vi "Stage Double Click.vi"(7 "Draw Area Size":T1, 8 "error in (no error)":errorcluster, 9 "Y (px)":i32, 10 "X (px)":i32, 11 "Application in":refnum<class "Application.lvclass">) -> (0 "error out":errorcluster, 3 "Application out":refnum<class "Application.lvclass">)   [LabVIEW 2023, in "Application.lvlib" / "Application.lvclass"]
uses:
  Application.lvclass
  Application.lvclass/Application.ctl
  Hardware/Stage Controller Messages/Move From Double Click Msg/Move From Double Click Msg.lvclass/Move From Double Click Msg.ctl
  <vilib>/ActorFramework/Message Enqueuer/Message Enqueuer.lvclass/Message Enqueuer.ctl
  <vilib>/ActorFramework/Message Enqueuer/Enqueue.vi
  Hardware/Stage Controller Messages/Move From Double Click Msg/Move From Double Click Msg.lvclass
  C:/Program Files/National Instruments/LabVIEW 2023/vi.lib/ActorFramework/Message/Message.lvclass
  <vilib>/ActorFramework/Message Priority Queue/Priority Enqueue.vi
  <vilib>/Utility/miscctls.llb/LVBoundsTypeDef.ctl
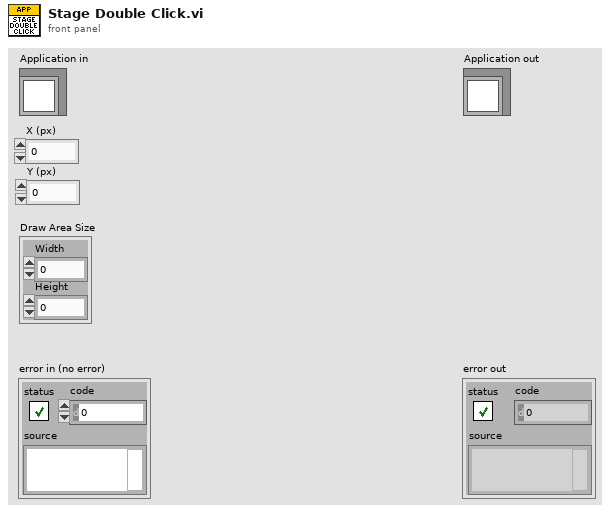
[diagram p1: front panel]
types:
  T1 = typedef "LVBoundsTypeDef.ctl" = cluster{"Width":u32, "Height":u32}
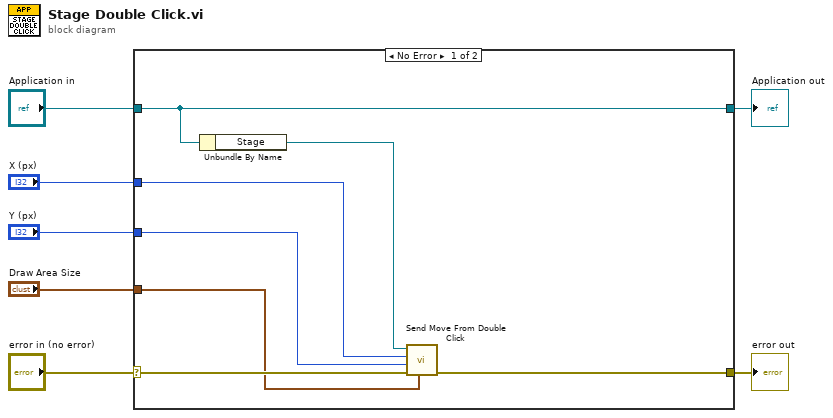
[diagram p0: block diagram]
diagram:
  n1 = case shown="No Error" "error in (no error)" {
    selector: "error in (no error)" -> [w13 w16]
    tunnel: [w12 w16] -> w6
    tunnel: [w14 w15] -> w4
    tunnel: "Application in" -> [w14 w15]
    tunnel: "X (px)" -> [w10 _]
    tunnel: "Y (px)" -> [w9 _]
    tunnel: "Draw Area Size" -> [w8 _]
    frame No Error {
      n2 = Unbundle By Name(w14) -> ("Stage"=w11:refnum<class "Message Enqueuer.lvclass">)
      n3 = call "Send Move From Double Click.vi"("Draw Area Size"=w8, "error in (no error)"=w13, "Y (px)"=w9, "X (px)"=w10, "Message Enqueuer"=w11) -> ("error out"=w12:errorcluster)  [unwired: 5 in, 1 out]
    }
    frame Error {
    }
  }
  "error out" <- w6
  "Application out" <- w4
